vi "Elapsed Time.vi"(9 "Reset Timer":bool, 10 "Target Time":dbl) -> (1 "Time Has Elapsed?":bool, 2 "Elapsed Time":dbl)   [LabVIEW 2016]
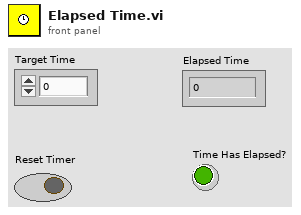
[diagram p1: front panel]
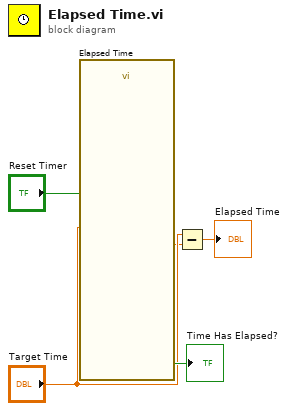
[diagram p0: block diagram]
diagram:
  n1 = call "Elapsed Time"("Time Target (s)"="Target Time", "Reset"="Reset Timer") -> ("Elapsed Time (s)"=w2:dbl, "Time has Elapsed"=→"Time Has Elapsed?":bool)  [unwired: 10 in, 6 out]
  n2 = Subtract(x="Target Time", y=w2) -> (x-y=→"Elapsed Time":dbl)
